vi "Save AOI list.vi"   [LabVIEW 2011]
doc: "Saves the global AOI list coordinates as a user-specified file. Note that the internal AOI list is in x1, y1, x2, y2 format whereas the file is converted into x, y, dx, dy format to preserved compatibility with other software."
uses:
  AOI List Globals.vi
  <vilib>/Utility/file.llb/Write To Spreadsheet File (I64).vi
types:
  T1 = enum16{"open", "open or create", "create or replace", "create"}
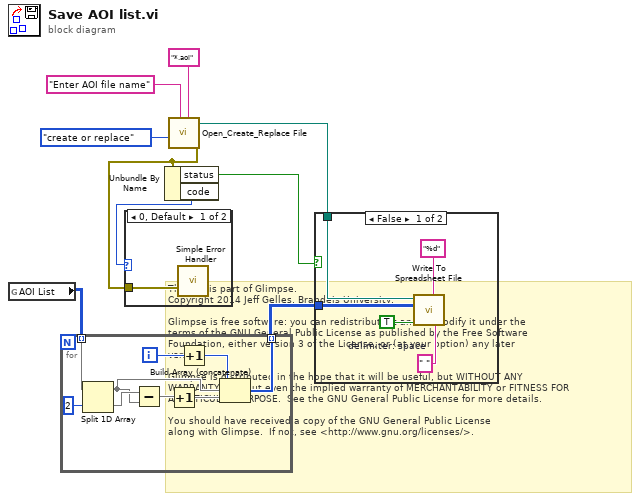
[diagram p0: block diagram]
diagram:
  # "This file is part of Glimpse. \nCopyright 2014 Jeff Gelles, Brandeis University.    \n\nGlimpse is free software: you can redistribute it and/or modify it under the \nterms of the GNU General Public License as published by the Free Software \nFoundation, either version 3 of the License, or (at your option) any later \nversion.\n\nGlimpse is distributed in the hope that it will be useful, but WITHOUT ANY \nWARRANTY; without even the implied warranty of MERCHANTABILITY or FITNESS FOR \nA PARTICULAR PURPOSE.  See the GNU General Public License for more details.\n\nYou should have received a copy of the GNU General Public License\nalong with Glimpse.  If not, see <http://www.gnu.org/licenses/>."
  n1 = global read "AOI List Globals.vi" "AOI List"() -> (w9:u16[][])
  n2 = for {
    tunnel: w9 -> [w18] mode=indexing
    tunnel: [w12] -> w8 mode=indexing
    i -> [w11]
    n3 = Split 1D Array(array=w18, index=2) -> (first subarray=w13:u16[], second subarray=w16:u16[])
    n4 = Subtract(x=w16, y=w13) -> (x-y=w15:u16[])
    n5 = Increment(x=w15) -> (x+1=w14:u16[])
    n6 = Increment(x=w11) -> (x+1=w10:i32)
    n7 = Build Array (concatenate)(w10, w13, w14) -> (w12:i32[])
  }
  n8 = call <vilib>:"Open_Create_Replace File.vi"("pattern"="*.aoi", "prompt"="Enter AOI file name", "function (open:0)"=T1."create or replace") -> ("error out"=w6:errorcluster, "new file path"=w4:path)  [unwired: 4 in, 3 out]
  n9 = Unbundle By Name(w6) -> ("status"=w5:bool, "code"=w7:i32)
  n10 = case shown="0, Default" w7 {
    tunnel: w6 -> [w19 _]
    frame 0, Default {
      n11 = call <vilib>:"Simple Error Handler.vi"("error in (no error)"=w19) -> ()  [unwired: 1 in, 8 out]
    }
    frame 43 {
    }
  }
  n12 = case shown="False" w5 {
    tunnel: w8 -> [w22 _]
    tunnel: w4 -> [w21 _]
    frame False {
      w24 = " "  # delimiter: space
      n13 = call-poly <vilib>:"Write To Spreadsheet File.vi"("delimiter (\\t)"=w24, "format (%d)"="%d" ("format (%.3f)"), "append to file? (new file:F)"=TRUE, "2D data"=w22, "file path (dialog if empty)"=w21) -> ()  [unwired: 2 in, 2 out]
    }
    frame True {
    }
  }
